vi "LogSingleTone.vi"(5 "MaxValue":sgl[](array[numeric]), 6 "LogTime?":bool, 8 "error in":errorcluster, 9 "seconds since 1Jan1904":timestamp[](array[timestamp]), 10 "Cal":T1 {"Downshift_dset" format="%.0x"; "DeltaPhase_dset" format="%.0x"; "Phase_dset" format="%.0x"; "SNR_dset" format="%.0x"; "df_dset" format="%.0x"; "PeakLoc_dset" format="%.0x"; "MaxValue_dset" format="%.0x"; "TImeStamp_dset" format="%.0x"; "TimeString_dset" format="%.0x"}) -> (0 "error out":errorcluster)   [LabVIEW 2018]
uses:
  HDF5_Tone_refs.ctl
  <vilib>/addons/h5labview2/base/hid_t.ctl
  lib_path_mod_20200519.vi
  <vilib>/addons/h5labview2/base/H5Equery.vi
  <vilib>/addons/h5labview2/dataset/H5Dwrite.llb/H5Dwrite.xnode
  <vilib>/addons/h5labview2/dataset/H5D.lvlib
  <vilib>/addons/h5labview2/space/H5S.lvlib
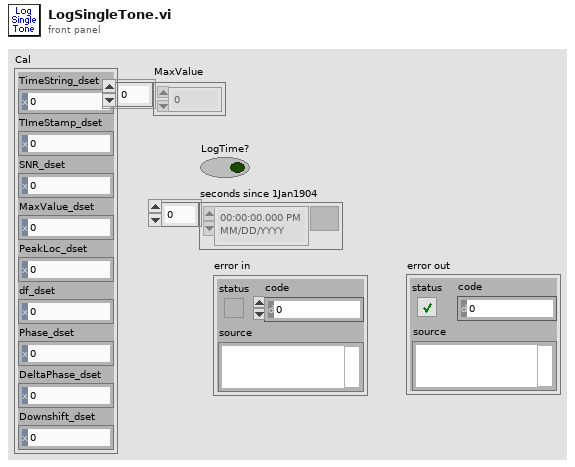
[diagram p1: front panel]
types:
  T1 = typedef "HDF5_Tone_refs.ctl" = cluster{"TimeString_dset":T2, "TImeStamp_dset":T2, "SNR_dset":T2, "MaxValue_dset":T2, "PeakLoc_dset":T2, "df_dset":T2, "Phase_dset":T2, "DeltaPhase_dset":T2, "Downshift_dset":T2}
  T2 = typedef "hid_t.ctl" = i32
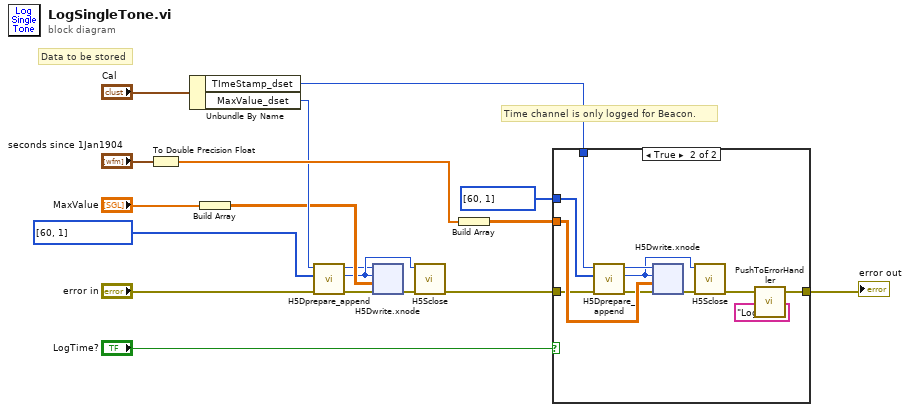
[diagram p0: block diagram]
diagram:
  # "Time channel is only logged for Beacon."
  # "Data to be stored"
  n1 = To Double Precision Float(number="seconds since 1Jan1904") -> (double precision float=w18:dbl[])
  n2 = Unbundle By Name("Cal") -> ("TImeStamp_dset"=w17:T2, "MaxValue_dset"=w13:T2)
  n3 = Build Array("MaxValue") -> (w10:sgl[][])
  n4 = call <vilib>:"H5Dprepare_append.vi"("error in (no error)"="error in", "append dims"=u64[] [60, 1], "dset in"=w13) -> ("error out"=w7:errorcluster, "space out"=w9:T2, "dset out"=w8:T2)  [unwired: 5 in, 1 out]
  n5 = xnode "H5Dwrite.xnode"("error in (no error)"=w7, "data"=w10, "file space"=w9, "ref in"=w8) -> ("error out"=w6:errorcluster)  [unwired: 3 in, 2 out]
  n6 = call <vilib>:"H5Sclose.vi"("error in (no error)"=w6, "space in"=w9) -> ("error out"=w3:errorcluster)  [unwired: 9 in]
  n7 = Build Array(w18) -> (w12:dbl[][])
  n8 = case shown="True" "LogTime?" {
    tunnel: w17 -> [_ w30]
    tunnel: [w19 w29] -> w15
    tunnel: w12 -> [_ w28]
    tunnel: u64[] [60, 1] ("append dims") -> [_ w23]
    tunnel: w3 -> [w19 w22]
    frame False {
    }
    frame True {
      n9 = call <vilib>:"H5Dprepare_append.vi"("error in (no error)"=w22, "append dims"=w23, "dset in"=w30) -> ("error out"=w26:errorcluster, "space out"=w24:T2, "dset out"=w25:T2)  [unwired: 5 in, 1 out]
      n10 = xnode "H5Dwrite.xnode"("error in (no error)"=w26, "data"=w28, "file space"=w24, "ref in"=w25) -> ("error out"=w27:errorcluster)  [unwired: 3 in, 2 out]
      n11 = call <vilib>:"H5Sclose.vi"("error in (no error)"=w27, "space in"=w24) -> ("error out"=w21:errorcluster)  [unwired: 9 in]
      n12 = call "PushToErrorHandler.vi"("ErrorIn"=w21, "ErrorLocation"="LogTime") -> ("ErrorOut"=w29:errorcluster)  [unwired: 5 in]
    }
  }
  "error out" <- w15
